vi "Kaelus PIM SetTxPwr TCP Cmds.vi"(4 "Legacy (f)?":bool, 6 "Force?":bool, 8 "error in":errorcluster, 9 "Carrier Powers":cluster{"C1 Power,dBm":dbl, "C2 Power, dBm":dbl}) -> (0 "error out":errorcluster)   [LabVIEW 2011]
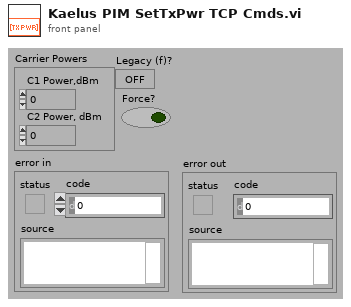
[diagram p1: front panel]
types:
  T1 = typedef "PIM.API.Command.Unique.ctl" = cluster{"#attributes":cluster{"Action":string}, "Double":dbl[], "Integer":i32[], "Boolean":bool[], "String":string[]}
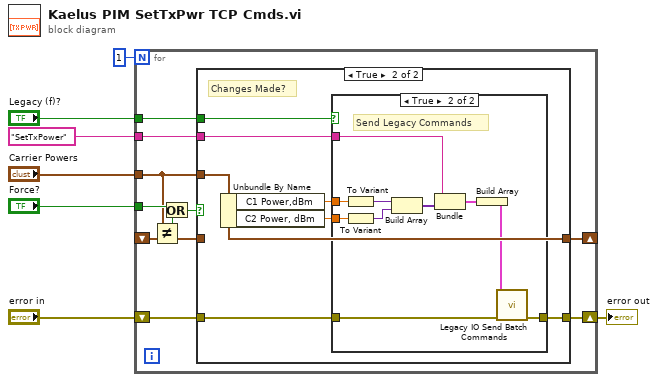
[diagram p0: block diagram]
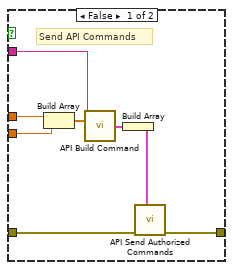
[diagram p3: hidden frame]
diagram:
  n1 = for {
    N: 1 -> [_]
    tunnel: "SetTxPower" -> [w15]
    tunnel: "Legacy (f)?" -> [w14]
    tunnel: "Force?" -> [w11]
    tunnel: "Carrier Powers" -> [w10]
    shift-right: [w16] -> w3
    shift-left: "error in" -> [w17]
    shift-right: [w9] -> _
    shift-left: _ -> [w8]
    n2 = Not Equal?(x=w10, y=w8) -> (x != y?=w12:bool)
    n3 = Or(x=w11, y=w12) -> (x .or. y?=w13:bool)
    n4 = case shown="True" w13 {
      tunnel: w10 -> [_ w20]
      tunnel: w17 -> [w19 w24]
      tunnel: [w19 w23] -> w16
      tunnel: w15 -> [_ w22]
      tunnel: w14 -> [_ w21]
      tunnel: [w18 w20] -> w9
      tunnel: w8 -> [w18 _]
      frame False {
        # "No Changes were made"
      }
      frame True {
        # "Changes Made?"
        n5 = Unbundle By Name(w20) -> ("C1 Power,dBm"=w26:dbl, "C2 Power, dBm"=w25:dbl)
        n6 = case shown="True" w21 {
          tunnel: w26 -> [w34 w43]
          tunnel: w25 -> [w33 w42]
          tunnel: w24 -> [w28 w37]
          tunnel: [w27 w36] -> w23
          tunnel: w22 -> [w31 w35]
          frame False {
            # "Send API Commands"
            n7 = Build Array(w34, w33) -> (w32:dbl[])
            n8 = call "API Build Command.vi"("Action"=w31, "Double"=w32) -> ("PIM.API.Command.Unique"=w30:T1)  [unwired: 13 in]
            n9 = Build Array(w30) -> (w29:T1[])
            n10 = call "API Send Authorized Commands.vi"("Commands"=w29, "error in (no error)"=w28) -> ("error out"=w27:errorcluster)  [unwired: 7 in, 2 out]
          }
          frame True {
            # "Send Legacy Commands"
            n11 = To Variant(anything=w43) -> (Variant=w41:variant)
            n12 = To Variant(anything=w42) -> (Variant=w40:variant)
            n13 = Build Array(w41, w40) -> (w39:variant[])
            n14 = Bundle(w35, w39) -> (w44:cluster{string, variant[]})  [unwired: 1 out]
            n15 = Build Array(w44) -> (w38:cluster{string, variant[]}[])
            n16 = call "Legacy IO Send Batch Commands.vi"("error in"=w37, "Legacy Commands Array"=w38) -> ("error out"=w36:errorcluster)  [unwired: 9 in]
          }
        }
      }
    }
  }
  "error out" <- w3
